vi "Read_USB.vi"(8 "entrée d'erreur (pas d'erreur)":errorcluster, 10 "timeout (0)":u32, 11 "Nom de ressource VISA":refnum<visa-resource-name>) -> (0 "sortie d'erreur":errorcluster, 1 "chaîne en sortie":string, 3 "Nom de ressource VISA en sortie":refnum<visa-resource-name>)   [LabVIEW 2013]
uses:
  <vilib>/Instr/_visa.llb/Select Event Type.ctl
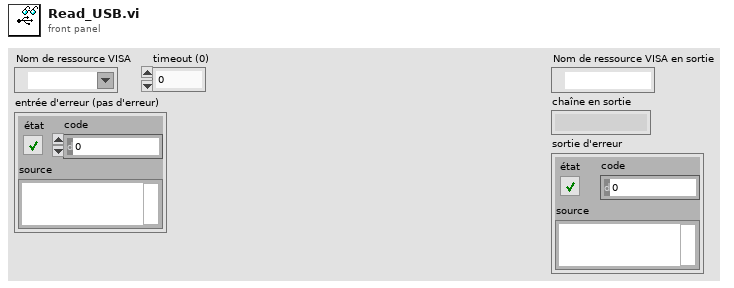
[diagram p1: front panel]
types:
  T1 = typedef "Select Event Type.ctl" = u32
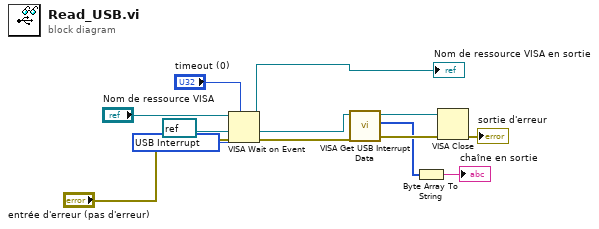
[diagram p0: block diagram]
diagram:
  w11 = T1 1073684535 items=["Service Request"=1073684491, "Trigger"=3221168138, "Clear"=1073684493, "VXI Signal"=1073684512, "VXI/VME Interrupt"=3221168161, "VXI/VME Sysfail"=1073684509, "VXI/VME Sysreset"=1073684510, "GPIB-CIC"=1073684498, "GPIB-Talk"=1073684499, "GPIB-Listen"=1073684500, "PXI Interrupt"=1073684514, "Serial Break"=1073684515, "Serial TermChar"=1073684516, "Serial CTS"=1073684521, "Serial DSR"=1073684522, "Serial DCD"=1073684524, "Serial RI"=1073684526, "Serial Character"=1073684533, "USB Interrupt"=1073684535, "All Enabled"=1073709055] ("Event Type")
  n1 = VISA Wait on Event(7:"timeout (0)", 8:"entrée d'erreur (pas d'erreur)", 9:refnum<visa-resource-name> refnum ("VISA USB Intr Event"), 10:w11, 11:"Nom de ressource VISA") -> (0:w6:errorcluster, 1:w7:refnum<visa-resource-name>, 3:→"Nom de ressource VISA en sortie":refnum<visa-resource-name>)  [unwired: 1 out]
  n2 = call <vilib>:"VISA Get USB Interrupt Data.vi"("error in (no error)"=w6, "VISA USB Intr Event"=w7) -> ("error out"=w4:errorcluster, "data buffer"=w3:u8[], "VISA USB Intr Event out"=w5:refnum<visa-resource-name>)  [unwired: 7 in]
  n3 = Byte Array To String(unsigned byte array=w3) -> (string=→"chaîne en sortie":string)
  n4 = VISA Close(VISA resource name=w5, error in (no error)=w4) -> (error out=→"sortie d'erreur":errorcluster)
